vi "Quit.vi"(0 "Notifier Name":string, 11 "Error In":errorcluster) -> (4 "Notifier Name Dup":string, 15 "Error Out":errorcluster)   [LabVIEW 2020]
uses:
  3 Mirror Scan Type Defs/3 Mirror Scan Note Type.ctl
  3 Mirror Scan Type Defs/3 Mirror Scan Actions.ctl
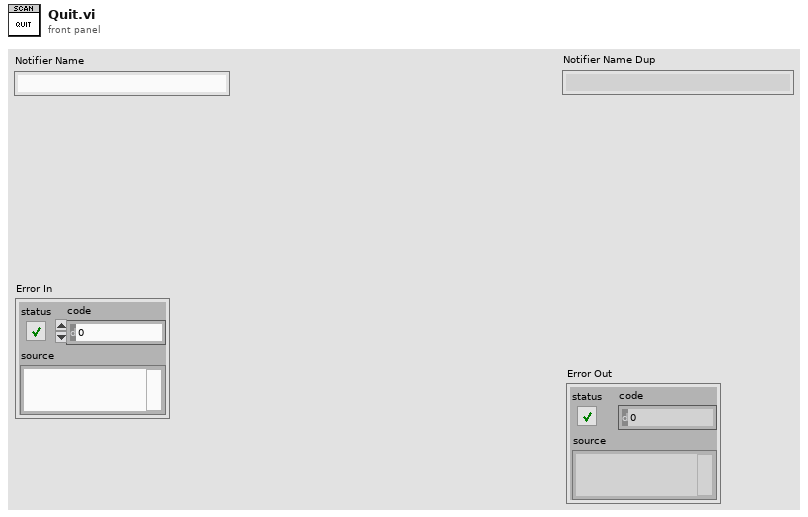
[diagram p1: front panel]
types:
  T1 = typedef "3 Mirror Scan Note Type.ctl" = cluster{"Actions":T2, "Global Rectangle":i32[], "Running":bool, "Scan Frequency (Hz)":dbl, "Scan Time (s)":dbl}
  T2 = typedef "3 Mirror Scan Actions.ctl" = enum16{"Idle", "Scan Timed", "Scan Live", "Convert ROI", "Run Scan", "Exit Loop", "Quit"}
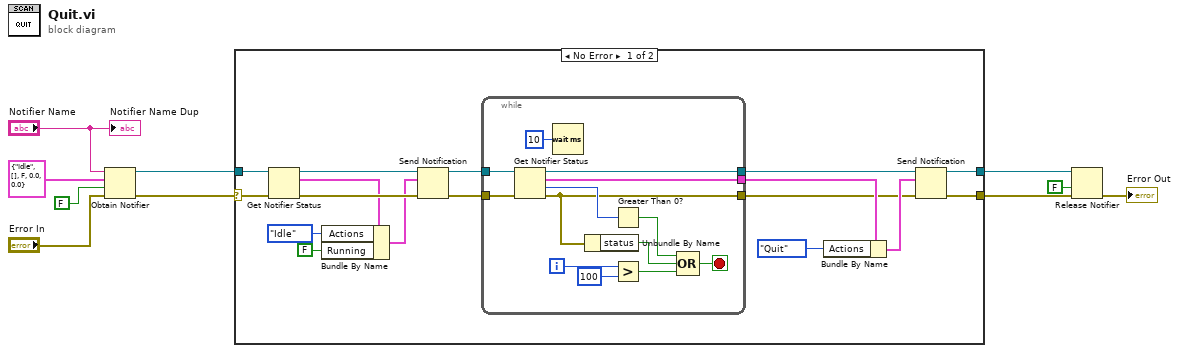
[diagram p0: block diagram]
diagram:
  n1 = Obtain Notifier(name (unnamed)="Notifier Name", notification data type=T1 {"Actions"=enum."Idle", "Global Rectangle"=[], "Running"=FALSE, "Scan Frequency (Hz)"=0.0, "Scan Time (s)"=0.0} ("3 Mirror Notifier"), create if not found? (T)=FALSE, error in (no error)="Error In") -> (notifier out=w6:refnum<notifier>, error out=w7:errorcluster)  [unwired: 1 out]
  n2 = case shown="No Error" w7 {
    selector: w7 -> [w26 w41]
    tunnel: w6 -> [w27 w42]
    tunnel: [w12 w42] -> w4
    tunnel: [w11 w41] -> w2
    frame No Error {
      n3 = Get Notifier Status(notifier=w27, error in (no error)=w26) -> (notifier out=w25:refnum<notifier>, current notification=w23:T1, error out=w24:errorcluster)  [unwired: 2 out]
      n4 = Bundle By Name(cluster=w23, "Actions"=3_Mirror_Scan_Actions."Idle", "Running"=FALSE) -> (w20:T1)
      n5 = Send Notification(notification=w20, notifier=w25, error in (no error)=w24) -> (notifier out=w19:refnum<notifier>, error out=w18:errorcluster)
      n6 = while {
        tunnel: w19 -> [w40]
        tunnel: w18 -> [w39]
        tunnel: [w31] -> w17
        tunnel: [w30] -> w13
        tunnel: [w28] -> w14
        i -> [w37]
        stop <- w32 stop-if-true
        n7 = Get Notifier Status(notifier=w40, error in (no error)=w39) -> (notifier out=w31:refnum<notifier>, current notification=w28:T1, # waiting=w35:i32, error out=w30:errorcluster)  [unwired: 1 out]
        n8 = Wait (ms)(milliseconds to wait=u32 10) -> ()  [unwired: 1 out]
        n9 = Unbundle By Name(w30) -> ("status"=w34:bool)
        n10 = Greater Than 0?(x=w35) -> (x > 0?=w29:bool)
        n11 = Greater?(x=w37, y=100) -> (0:w33:bool)
        n12 = Compound Arithmetic op=OR(w29, w34, w33) -> (w32:bool)
      }
      n13 = Bundle By Name(cluster=w14, "Actions"=3_Mirror_Scan_Actions."Quit") -> (w15:T1)
      n14 = Send Notification(notification=w15, notifier=w17, error in (no error)=w13) -> (notifier out=w12:refnum<notifier>, error out=w11:errorcluster)
    }
    frame Error {
    }
  }
  n15 = Release Notifier(notifier=w4, force destroy? (F)=FALSE, error in (no error)=w2) -> (error out=→"Error Out":errorcluster)  [unwired: 2 out]
  "Notifier Name Dup" <- "Notifier Name"
